vi "ref_is_valid.vi"(8 "error in (no error)":errorcluster, 11 "Item in":refnum<class "Item.lvclass">) -> (0 "error out":errorcluster, 2 "ref_is_valid?":bool, 3 "Item out":refnum<class "Item.lvclass">)   [LabVIEW 2020, in "toml_edit.lvlib" / "Item.lvclass"]
uses:
  Item.lvclass
  Item.lvclass/Item.ctl
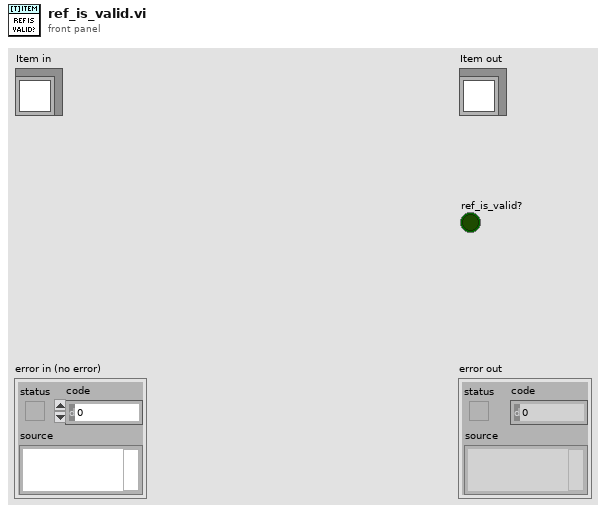
[diagram p1: front panel]
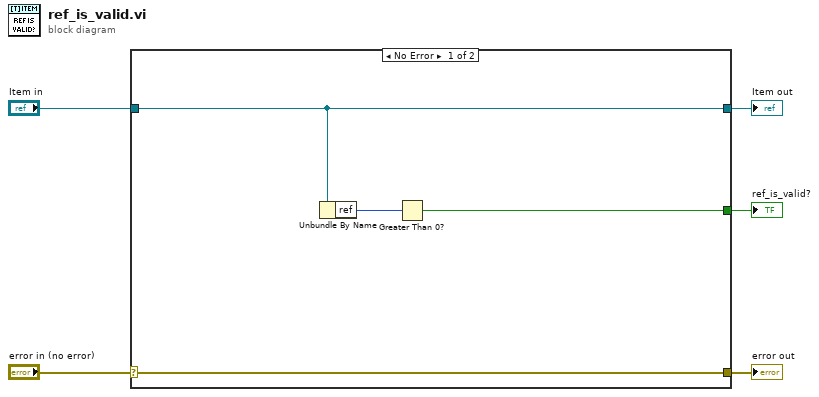
[diagram p0: block diagram]
diagram:
  n1 = case shown="No Error" "error in (no error)" {
    selector: "error in (no error)" -> [w9 w11]
    tunnel: [w9 w11] -> w4
    tunnel: [w8 w10] -> w2
    tunnel: "Item in" -> [w8 w10]
    tunnel: [w6 _] -> w1
    frame No Error {
      n2 = Unbundle By Name(w8) -> ("ref"=w7:u64)
      n3 = Greater Than 0?(x=w7) -> (x > 0?=w6:bool)
    }
    frame Error {
    }
  }
  "error out" <- w4
  "Item out" <- w2
  "ref_is_valid?" <- w1
